vi "sound.vi"(3 "frequency":dbl=10.0 format="%0.2p") -> ()   [LabVIEW 2014]
uses:
  <vilib>/sound2/lvsound2.llb/Sound Data Format.ctl
  <vilib>/sound2/lvsound2.llb/Sound Output Set Volume (Single).vi
  <vilib>/sound2/lvsound2.llb/Sound Output Write (DBL Single).vi
  <vilib>/measure/NI_MABase.lvlib
panel:
  in  "volume":dbl=100.0
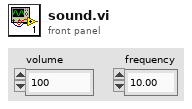
[diagram p1: front panel]
types:
  T1 = typedef "Sound Data Format.ctl" = cluster{"sample rate (S/s)":dbl, "number of channels":i32, "bits per sample":i32}
  T2 = typedef "Sound Output Task ID.ctl" = u32
  T3 = cluster{"sample rate (S/s)":dbl, "number of samples/ch":i32}
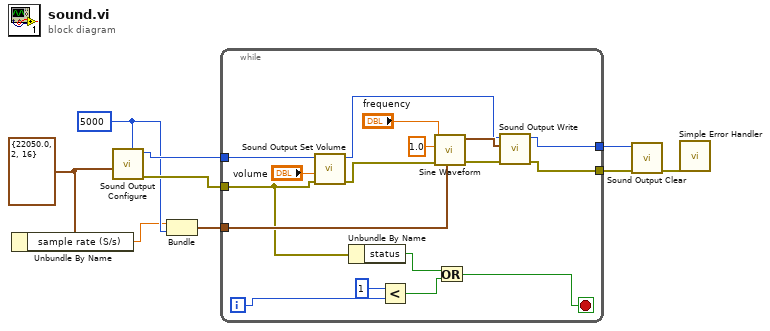
[diagram p0: block diagram]
diagram:
  w6 = 5000 ("number of samples/ch")
  w7 = T1 {"sample rate (S/s)"=22050.0, "number of channels"=2, "bits per sample"=16} ("sound format")
  n1 = Unbundle By Name(w7) -> ("sample rate (S/s)"=w5:dbl)
  n2 = call <vilib>:"Sound Output Configure.vi"("number of samples/ch"=w6, "sound format"=w7) -> ("error out"=w8:errorcluster, "task ID"=w9:T2)  [unwired: 8 in]
  n3 = Bundle("sample rate (S/s)"=w5, "number of samples/ch"=w6) -> (w4:T3)  [unwired: 1 in]
  n4 = while {
    tunnel: w9 -> [w24]
    tunnel: w8 -> [w15]
    tunnel: w4 -> [w19]
    tunnel: [w17] -> w3
    tunnel: [w16] -> w2
    i -> [w14]
    stop <- w10 stop-if-true
    n5 = call-poly <vilib>:"Sound Output Set Volume.vi"("error in (no error)"=w15, "volume"="volume", "task ID"=w24) -> ("error out"=w23:errorcluster, "task ID out"=w18:T2)  [unwired: 7 in]
    n6 = Unbundle By Name(w15) -> ("status"=w12:bool)
    n7 = Less?(x=1, y=w14) -> (x < y?=w11:bool)
    n8 = call <vilib>:"Sine Waveform.vi"("sampling info"=w19, "error in (no error)"=w23, "amplitude"=1.0, "frequency"="frequency") -> ("error out"=w21:errorcluster, "signal out"=w22:waveform(dbl))  [unwired: 6 in]
    n9 = Or(x=w12, y=w11) -> (x .or. y?=w10:bool)
    n10 = call-poly <vilib>:"Sound Output Write.vi"("error in (no error)"=w21, "data"=w22, "task ID"=w18) -> ("error out"=w16:errorcluster, "task ID out"=w17:T2)  [unwired: 7 in]
  }
  n11 = call <vilib>:"Sound Output Clear.vi"("error in (no error)"=w2, "task ID"=w3) -> ("error out"=w1:errorcluster)  [unwired: 9 in]
  n12 = call <vilib>:"Simple Error Handler.vi"("error in (no error)"=w1) -> ()  [unwired: 4 in, 5 out]
